vi "1553 Address Handles to Write Info.vi"(8 "error in":errorcluster, 11 "Address Based Execution Unit Implementation in":refnum<class "Address Based Execution Unit.lvclass">) -> (0 "error out":errorcluster, 3 "Address Based Execution Unit Implementation out":refnum<class "Address Based Execution Unit.lvclass">)   [LabVIEW 2020, in "Ballard MIL-STD-1553 Engine.lvlib" / "Implementation.lvlib" / "Address Based Execution Unit.lvclass"]
uses:
  Address Based Execution Unit.lvclass
  C:/dev/niveristand-ballard-milStd1553-custom-device/Source/Custom Device Support/Engine/Implementation/Execution Unit/Execution Unit.lvclass
  Address Write Info.ctl
  Shared/Address.ctl
  Acyclic Trigger Info.ctl
  Execution Unit/Execution Unit.lvclass/Execution Unit.ctl
  Address Based Execution Unit.lvclass/Address Based Execution Unit.ctl
  <instrlib>/BTI1553Lib/BTI1553LV.lvlib
  Execution Unit/Execution Unit.lvclass
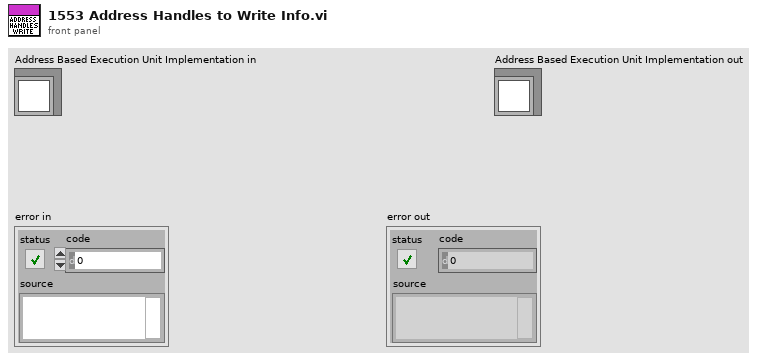
[diagram p1: front panel]
types:
  T1 = typedef "Ballard MIL-STD-1553 Engine.lvlib/Implementation.lvlib/Address Based Execution Unit.lvclass/Acyclic Trigger Info.ctl" = cluster{"bus controller handle":u64, "name":string}
  T2 = typedef "Ballard MIL-STD-1553 Engine.lvlib/Implementation.lvlib/Address Based Execution Unit.lvclass/Address Write Info.ctl" = cluster{"terminal address":T3, "terminal handle":u64}
  T3 = typedef "Address.ctl" = u16
  T4 = typedef "Ballard MIL-STD-1553 Engine.lvlib/Implementation.lvlib/Address Based Execution Unit.lvclass/1553 Address Based Handles.ctl" = cluster{"start stop handles":T5[], "acyclic frame trigger handles":T7[]}
  T5 = typedef "Ballard MIL-STD-1553 Engine.lvlib/Implementation.lvlib/Address Based Execution Unit.lvclass/Start Stop Channel Handles.ctl" = cluster{"terminal address":T3, "start handle":T6, "stop handle":T6}
  T6 = typedef "Custom Device API.lvlib/Custom Device Item Ref.ctl" = u64
  T7 = typedef "Ballard MIL-STD-1553 Engine.lvlib/Implementation.lvlib/Address Based Execution Unit.lvclass/Acyclic Frame Trigger Handle.ctl" = cluster{"name":string, "handle":T6}
  T8 = typedef "Ballard MIL-STD-1553 Engine.lvlib/Custom Device.lvlib/Hardware Handles.ctl" = cluster{"core handle":u64, "core reader handle":u64, "channel handles":u64[]}
  T9 = typedef "1553 Channel.ctl" = cluster{"HW channel":u16, "terminals":T10[], "messages":T11[], "acyclic frame names":string[]}
  T10 = typedef "Terminal Name and Address.ctl" = cluster{"name":string, "terminal address":T3}
  T11 = typedef "Message Definition.ctl" = cluster{"name":string, "message type":T12, "endpoint Rx":T13, "endpoint Tx":T13, "mode code":u16, "number of words":u16, "parameters":cluster{"name":string, "default value":dbl, "unit":string, "parameter definition":T14}[], "create timestamp channel":bool}
  T12 = typedef "Message Type.ctl" = string
  T13 = typedef "Terminal Endpoint.ctl" = cluster{"terminal address":T3, "subaddress":T3}
  T14 = typedef "Parameter Definition.ctl" = cluster{"start index":i32, "size (bits)":i32, "encoding":enum16{"BNR", "BCD", "Discrete"}, "signed":bool, "multiplier":dbl, "offset":dbl}
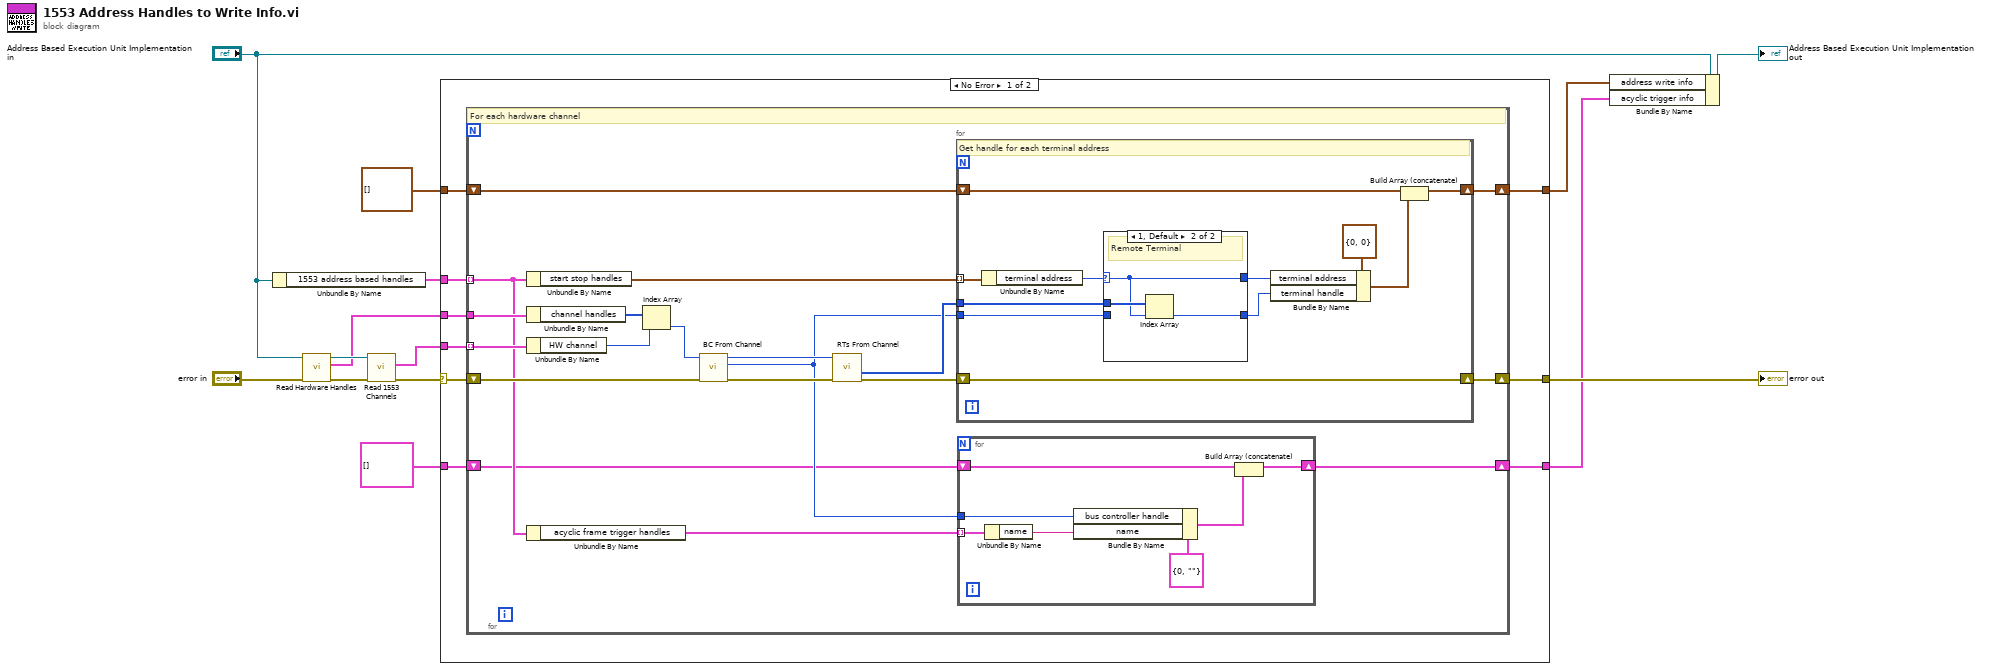
[diagram p0: block diagram]
diagram:
  n1 = Unbundle By Name("Address Based Execution Unit Implementation in") -> ("1553 address based handles"=w6:T4[])
  n2 = call "Read Hardware Handles.vi"("error in"="error in", "Execution Unit in"="Address Based Execution Unit Implementation in") -> ("error out"=w10:errorcluster, "hardware handles"=w7:T8, "Execution Unit out"=w8:refnum<class "Address Based Execution Unit.lvclass">)  [unwired: 7 in]
  n3 = call "Read 1553 Channels.vi"("error in"=w10, "Execution Unit in"=w8) -> ("error out"=w11:errorcluster, "1553 channels"=w12:T9[])  [unwired: 7 in, 1 out]
  n4 = case shown="No Error" w11 {
    selector: w11 -> [w22 w66]
    tunnel: w12 -> [w19 _]
    tunnel: w7 -> [w23 _]
    tunnel: [w21 w66] -> w14
    tunnel: w6 -> [w20 _]
    tunnel: T2[] [] ("address write info") -> [w18 _]
    tunnel: [w17 _] -> w3
    tunnel: T1[] [] -> [w16 _]
    tunnel: [w15 _] -> w1
    frame No Error {
      n5 = for {
        tunnel: w19 -> [w42] mode=indexing
        tunnel: w23 -> [w41]
        shift-right: [w36] -> w21
        shift-left: w22 -> [w32]
        tunnel: w20 -> [w28] mode=indexing
        shift-right: [w29] -> w17
        shift-left: w18 -> [w30]
        shift-right: [w24] -> w15
        shift-left: w16 -> [w25]
        # "For each hardware channel"
        n6 = Unbundle By Name(w28) -> ("start stop handles"=w35:T5[])
        n7 = Unbundle By Name(w41) -> ("channel handles"=w40:u64[])
        n8 = Unbundle By Name(w42) -> ("HW channel"=w39:u16)
        n9 = Unbundle By Name(w28) -> ("acyclic frame trigger handles"=w27:T7[])
        n10 = Index Array(array=w40, index=w39) -> (element=w34:u64)
        n11 = call <instrlib>:"BC From Channel.vi"("error in (no error)"=w32, "channel handle in"=w34) -> ("error out"=w31:errorcluster, "bus controller handle out"=w26:u64, "channel handle out"=w33:u64)  [unwired: 7 in]
        n12 = call <instrlib>:"RTs From Channel.vi"("error in (no error)"=w31, "channel handle in"=w33) -> ("error out"=w38:errorcluster, "remote terminal handles out"=w37:u64[])  [unwired: 6 in, 2 out]
        n13 = for {
          shift-right: [w60] -> w36
          shift-left: w38 -> [w60]
          tunnel: w37 -> [w58]
          tunnel: w35 -> [w59] mode=indexing
          tunnel: w26 -> [w56]
          shift-right: [w50] -> w29
          shift-left: w30 -> [w52]
          # "Get handle for each terminal address"
          n14 = Unbundle By Name(w59) -> ("terminal address"=w57:T3)
          n15 = case shown="1, Default" w57 {
            selector: w57 -> [w61 w63]
            tunnel: w58 -> [_ w65]
            tunnel: [w62 w64] -> w53
            tunnel: w56 -> [w62 _]
            tunnel: [w61 w63] -> w54
            frame 0 {
              # "Bus Controller"
            }
            frame 1, Default {
              # "Remote Terminal"
              n16 = Index Array(array=w65, index=w63) -> (element=w64:u64)
            }
          }
          n17 = Bundle By Name(cluster=T2 {"terminal address"=0, "terminal handle"=0} ("address write info"), "terminal address"=w54, "terminal handle"=w53) -> (w51:T2)
          n18 = Build Array (concatenate)(w52, w51) -> (w50:T2[])
        }
        n19 = for {
          tunnel: w27 -> [w49] mode=indexing
          tunnel: w26 -> [w45]
          shift-right: [w43] -> w24
          shift-left: w25 -> [w46]
          n20 = Unbundle By Name(w49) -> ("name"=w47:string)
          n21 = Bundle By Name(cluster=T1 {"bus controller handle"=0, "name"=""} ("acyclic trigger info"), "bus controller handle"=w45, "name"=w47) -> (w44:T1)
          n22 = Build Array (concatenate)(w46, w44) -> (w43:T1[])
        }
      }
    }
    frame Error {
    }
  }
  "error out" <- w14
  n23 = Bundle By Name(cluster="Address Based Execution Unit Implementation in", "address write info"=w3, "acyclic trigger info"=w1) -> (→"Address Based Execution Unit Implementation out":refnum<class "Address Based Execution Unit.lvclass">)
